vi "lua_settop.vi"(8 "error in (no error)":errorcluster, 10 "index":i32, 11 "lua_state_p":u64) -> (0 "error out":errorcluster, 3 "lua_state_p out":u64)   [LabVIEW 2020, in "lua.dll.lvlib"]
doc: "lua_settop\n[-?, +?, e]\nvoid lua_settop (lua_State *L, int index);\nAccepts any index, or 0, and sets the stack top to this index. If the new top is greater than the old one, then the new elements are filled with nil. If index is 0, then all stack elements are removed.\n\nThis function can run arbitrary code when removing an index marked as to-be-closed from the stack."
uses:
  lua.dll.lvlib
  lua54.dll
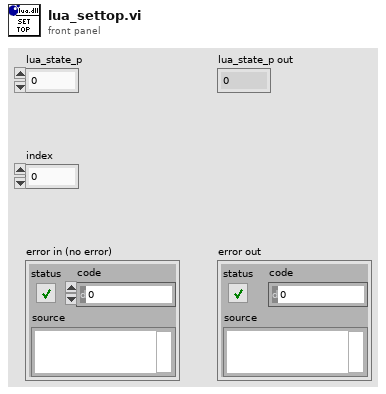
[diagram p1: front panel]
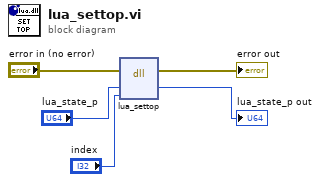
[diagram p0: block diagram]
diagram:
  n1 = dll-call lib="C:/Users/Nicholas Folse/Documents/workspace/github-tauterra.llc/Lua for LabVIEW/lib/lua.dll/lua54**.*" fn="lua_settop"(error in="error in (no error)", "lua_state_p"="lua_state_p", "index"="index") -> (error out=→"error out":errorcluster, "lua_state_p"=→"lua_state_p out":u64)  [unwired: 4 in, 1 out]
